vi "参数设置.vi"() -> (0 "设置完成的参数":T1={"frequency"=10.0, "amplitude"=1.0, "phase"=0.0, "sampling info"={"Fs"=1000.0, "#s"=1000.0}, "signal type"=0} {"signal type" items=["Sine Wave", "Triangle Wave", "Square Wave", "Sawtooth Wave"]; "sampling info"."Fs" format="%.2p"; "phase" format="%.2p"; "amplitude" format="%0.2p"; "frequency" format="%0.2p"})   [LabVIEW 2017]
panel:
  in  "设置":bool
  in  "参 数 设 置":T1={"frequency"=10.0, "amplitude"=1.0, "phase"=0.0, "sampling info"={"Fs"=1000.0, "#s"=1000.0}, "signal type"=0} {"signal type" items=["Sine Wave", "Triangle Wave", "Square Wave", "Sawtooth Wave"]; "sampling info"."Fs" format="%.2p"; "phase" format="%.2p"; "amplitude" format="%0.2p"; "frequency" format="%0.2p"}
  in  "取消":bool
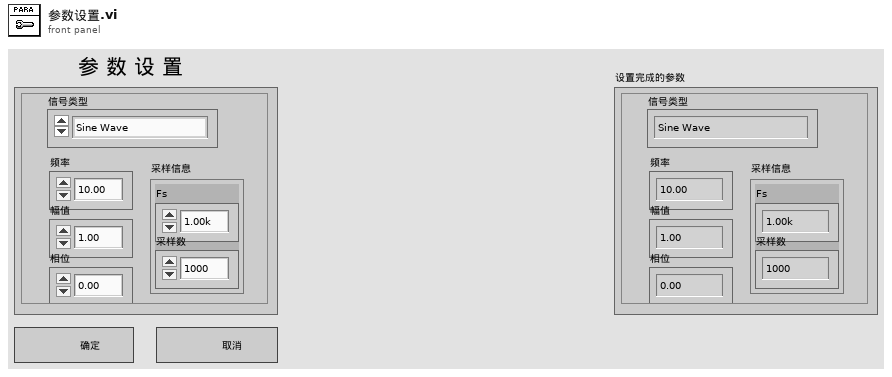
[diagram p1: front panel]
types:
  T1 = cluster{"frequency":dbl, "amplitude":dbl, "phase":dbl, "sampling info":cluster{"Fs":dbl, "#s":dbl}, "signal type":u16}
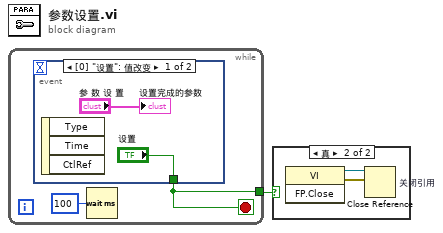
[diagram p0: block diagram]
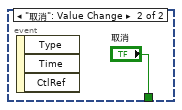
[diagram p3: hidden frame]
diagram:
  n1 = while {
    tunnel: [w2] -> w1
    stop <- w2 stop-if-true
    n2 = event shown="[0] \"设置\": 值改变" {
      selector: _ -> [_ _]
      dyn-events: _ -> [_ _]
      timeout: _ -> [_ _]
      tunnel: ["设置" "取消"] -> w2
      event "设置": Value Change {
        n3 = event-data() -> ()  [unwired: 1 in, 3 out]
        "设置完成的参数" <- "参 数 设 置"
      }
      event "取消": Value Change {
        n4 = event-data() -> ()  [unwired: 1 in, 3 out]
      }
    }
    n5 = Wait (ms)(milliseconds to wait=u32 100 ("等待时间（毫秒）")) -> ()  [unwired: 1 out]
  }
  n6 = case shown="真" w1 {
    frame False {
    }
    frame True {
      n7 = invoke class="VI" method="FP.Close"() -> (reference out=w8:refnum<vi>, error out=w7:errorcluster)  [unwired: 3 in, 1 out]
      n8 = Close Reference "关闭引用"(reference=w8, error in (no error)=w7) -> ()  [unwired: 1 out]
    }
  }
